vi "Check for passed test with given field data.vi"(6 "Optional where add on string in query":string, 7 "Part number":string="any", 8 "Error in (no error)":errorcluster, 9 "Got field?":bool=TRUE, 10 "Field data to check for":string, 11 "Field name":T1(ring)) -> (0 "Error out":errorcluster, 1 "RecordSet":string[][](array[string]), 2 "Records":i32, 3 "Passed rec with data?":bool)   [LabVIEW 2013]
doc: "Make part number = any if you don't want to use part number in search"
panel:
  out "final query":string
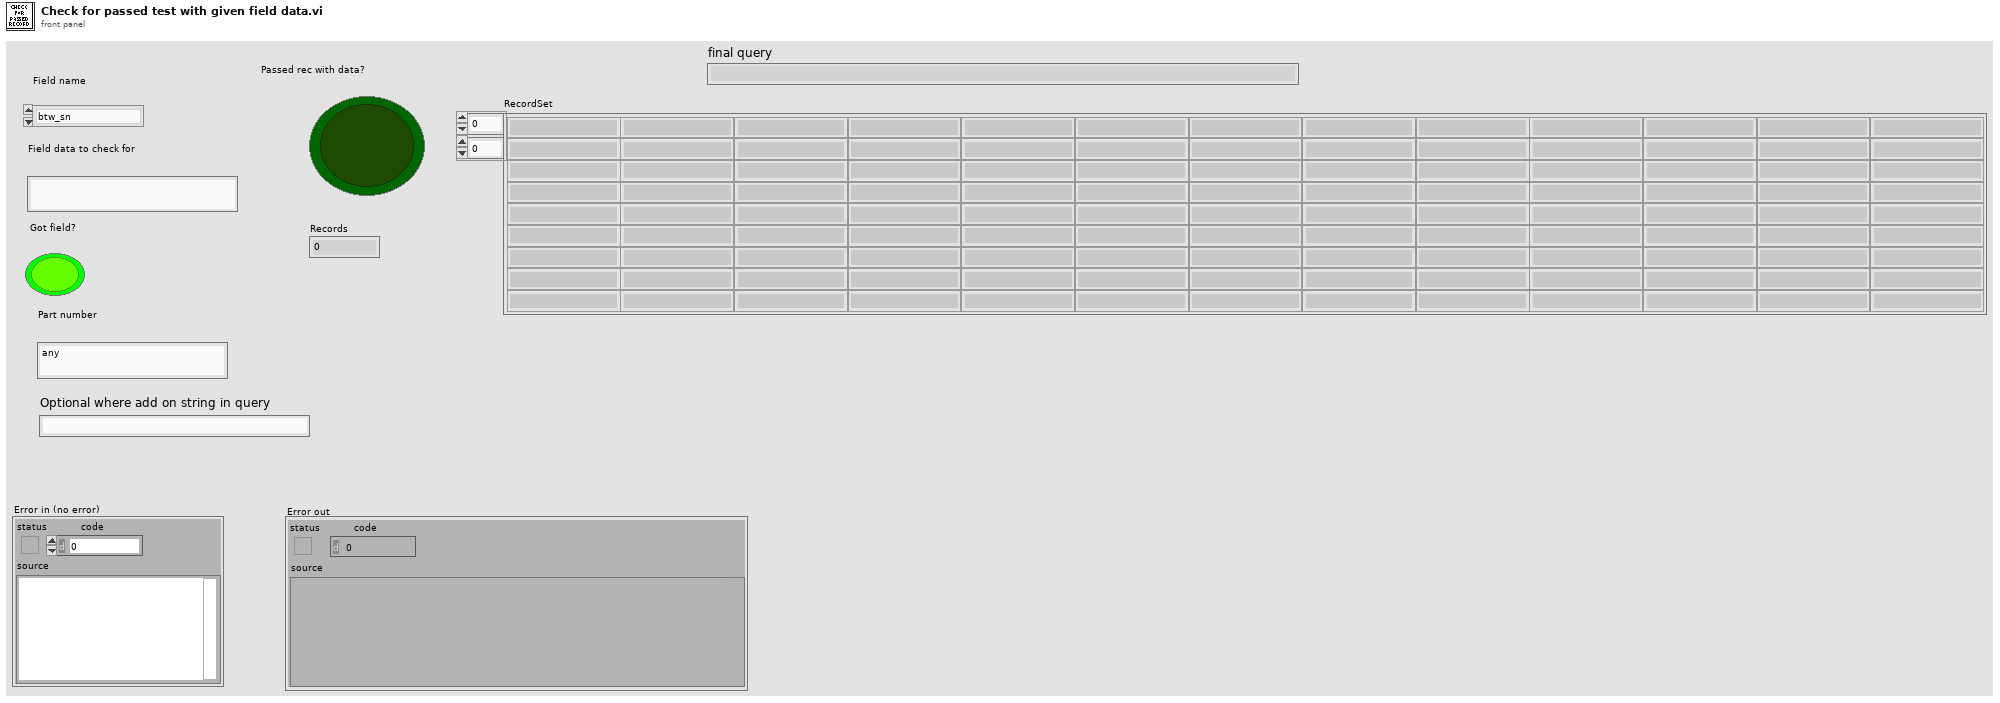
[diagram p1: front panel]
types:
  T1 = enum16{"btw_sn", "mac", "meid", "imei", "sim_id"}
  T2 = enum16{"Query", "Insert", "Select", "Dump Recs", "Get Rec Count", "Get Col Names", "Insert all fields", "Find", "Get last test result", "Get work order qty", "Set work order qty", "Save test report", "Get test report", "Execute query no data", "Select count", "Query and return row 0 col 0"}
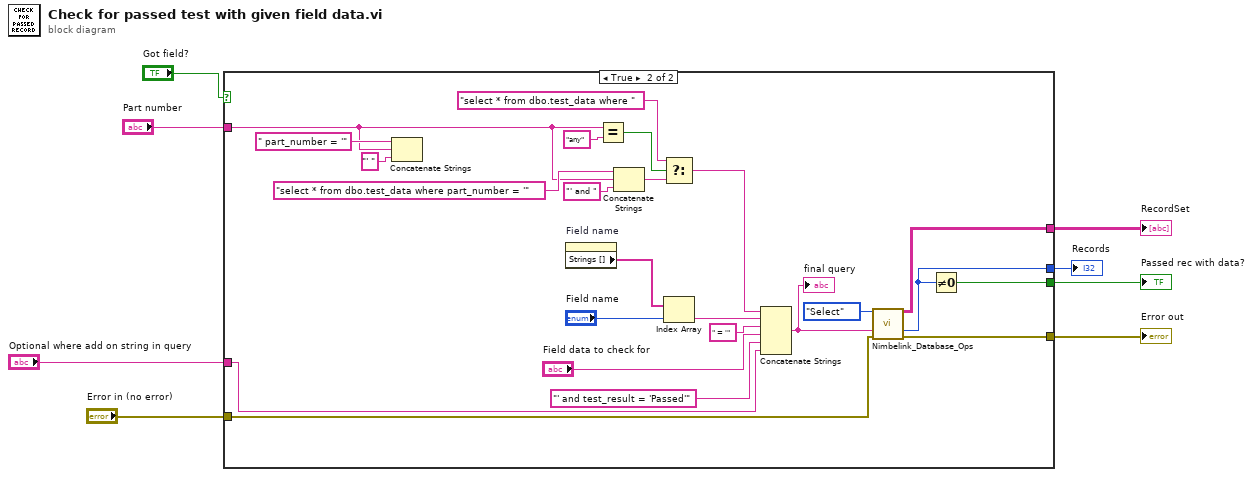
[diagram p0: block diagram]
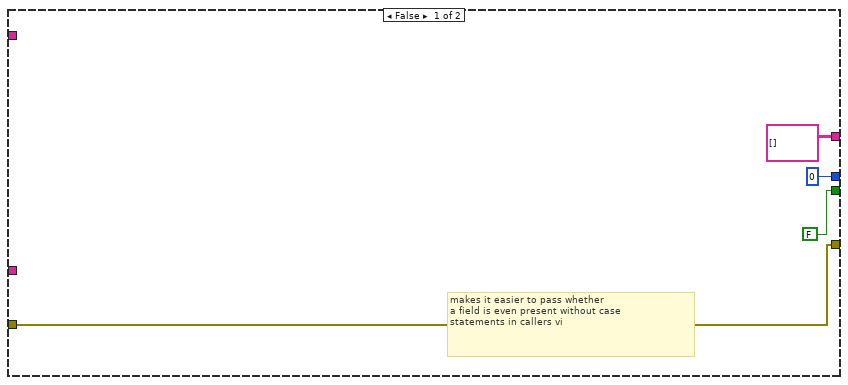
[diagram p2: hidden frame]
diagram:
  n1 = case shown="True" "Got field?" {
    tunnel: "Error in (no error)" -> [w11 w36]
    tunnel: [w11 w35] -> w7
    tunnel: [FALSE w26] -> w6
    tunnel: [0 ("Records") w25] -> w4
    tunnel: [string[][] [] ("RecordSet") w24] -> w3
    tunnel: "Part number" -> [_ w14]
    tunnel: "Optional where add on string in query" -> [_ w16]
    frame False {
      # "makes it easier to pass whether\na field is even present without case\nstatements in callers vi"
    }
    frame True {
      n2 = Concatenate Strings(" part_number = '", w14, "' " ("string")) -> ()  [unwired: 1 out]
      n3 = property on="Field name" class="Enum (strict)"() -> ("Strings []"=w32:string[])  [unwired: 2 in, 2 out]
      n4 = Equal?(x=w14, y="any") -> (x = y?=w22:bool)
      n5 = Concatenate Strings("select * from dbo.test_data where part_number = '", w14, "' and " ("string")) -> (w18:string)
      n6 = Select(t="select * from dbo.test_data where ", s=w22, f=w18) -> (s? t:f=w17:string)
      n7 = Index Array(array=w32, index="Field name") -> (element=w31:string)
      n8 = Concatenate Strings(w17, w31, " = '" ("string"), "Field data to check for", "' and test_result = 'Passed'" ("string"), w16) -> (w27:string)
      "final query" <- w27
      n9 = call "Nimbelink_Database_Ops.vi"("Operation"=T2."Select", "SQL Query"=w27, "Error in (no error)"=w36) -> ("RecordSet"=w24:string[][], "Records"=w25:i32, "Error out"=w35:errorcluster)  [unwired: 6 in, 4 out]
      n10 = Not Equal To 0?(x=w25) -> (x != 0?=w26:bool)
    }
  }
  "Error out" <- w7
  "Passed rec with data?" <- w6
  "Records" <- w4
  "RecordSet" <- w3
